vi "Find Element.vi"(8 "error in (no error)":errorcluster, 9 "Name":string, 11 "Variant (Cluster) in":variant) -> (0 "error out":errorcluster, 1 "index of element":i32, 2 "element":variant, 3 "Variant (Cluster) out":variant, 4 "found?":bool)   [LabVIEW 2017, in "Variant Data Manipulation.lvlib"]
uses:
  Variant Data Manipulation.lvlib
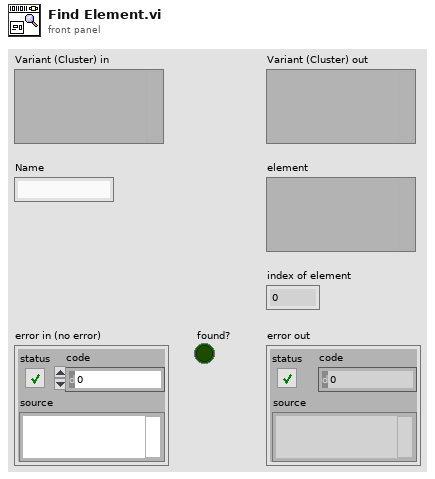
[diagram p1: front panel]
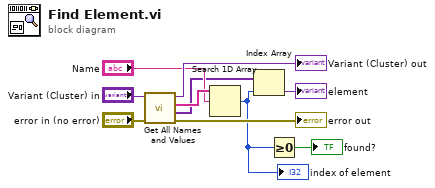
[diagram p0: block diagram]
diagram:
  n1 = call "Get All Names and Values.vi"("error in"="error in (no error)", "Cluster in"="Variant (Cluster) in") -> ("error out"=→"error out":errorcluster, "Values"=w5:variant[], "Element Names"=w8:string[], "Cluster out"=→"Variant (Cluster) out":variant)  [unwired: 5 in, 1 out]
  n2 = Search 1D Array(1D array=w8, element="Name") -> (index of element=w2:i32)  [unwired: 1 in]
  "index of element" <- w2
  n3 = Index Array(array=w5, index=w2) -> (element=→"element":variant)
  n4 = Greater Or Equal To 0?(x=w2) -> (x >= 0?=→"found?":bool)
